vi "R=Peg_In_Hole_Jig.vi"(8 "Offset":T3, 9 "Matrix":T2 format="%.3f", 11 "Command":string="Load") -> (0 "error out":errorcluster, 2 "Joints":dbl[](array[numeric]), 3 "Pose Out":T2 format="%.3f")   [LabVIEW 2013]
uses:
  <vilib>/Analysis/Matrix/Datatypes/RealMatrix.ctl
  ROS/Code/SubVIs/BaxterSide.ctl
  ROS/Code/Console/Servers/ServerSubs/(nist) Arm Globals.vi
  <vilib>/Utility/config.llb/Read Key (String).vi
  Arm Globals.vi
  <vilib>/Analysis/baseanly.llb/Real Inverse Matrix.vi
  <vilib>/Analysis/Matrix/Numeric/Multiply/Multiply - RM,RM.vi
  <vilib>/Analysis/Matrix/Numeric/Conversions/Array To Matrix - RA.vi
  <vilib>/Utility/config.llb/Write Key (String).vi
  <vilib>/Analysis/NI_AALBase.lvlib
  <vilib>/Analysis/Matrix/NI_Matrix.lvlib
  <vilib>/Utility/config.llb/NI_LVConfig.lvlib
panel:
  in  "Tab Control":T1(tab)=enum."Calibration Table"
  out "IK Found":bool=TRUE
  in  "Table":dbl[][](array[numeric])
  in  "Reference":dbl[](array[numeric])=[40.0, -60.0, 0.0, 65.0, 0.0, 70.0, 0.0]
  # "Basic Commands are:\n   Convert   - convert offset to joints\n   Current   - current joint and offset\n   Save      - save calibration data\n   Load      - load calibration data\n   Reference - give reference joint position"
  # "Object X       ObjectY         ObjectZ        ObjectA         BaseX           BaseY           BaseZ          BaseA"
  # "Far Left"
  # "Far Right"
  # "Near Left"
  # "Near Right"
  # "Create cfg file to maintain \ncalibration data.\n\nThese values are loaded from there."
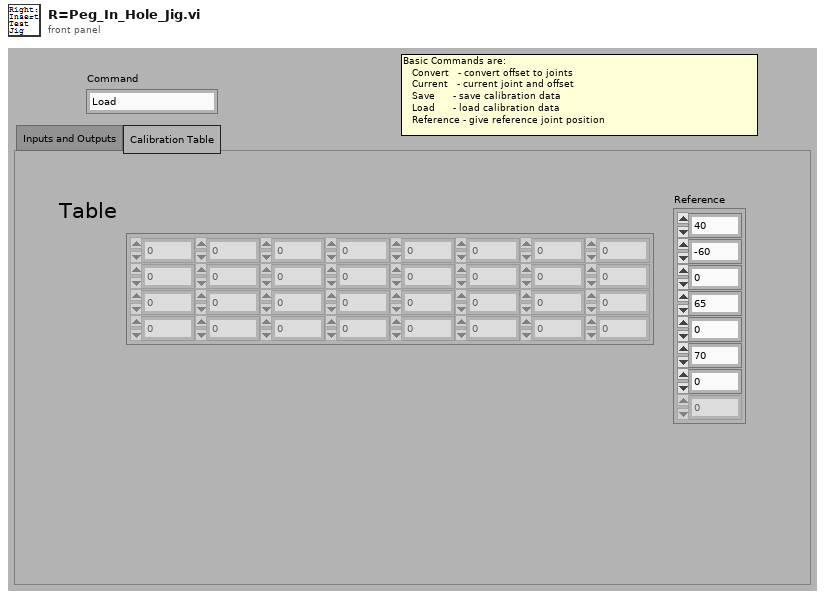
[diagram p1: front panel]
types:
  T1 = enum32{"Inputs and Outputs", "Calibration Table"}
  T2 = typedef "NI_Matrix.lvlib/RealMatrix.ctl" = dbl[][]
  T3 = cluster{"X":dbl, "Y":dbl, "Z":dbl, "Roll":dbl, "Pitch":dbl, "Yaw":dbl}
  T4 = typedef "BaxterSide.ctl" = enum16{"left", "right"}
  T5 = typedef "NI_LVConfig.lvlib/Config Data RefNum.ctl" = refnum<k1>
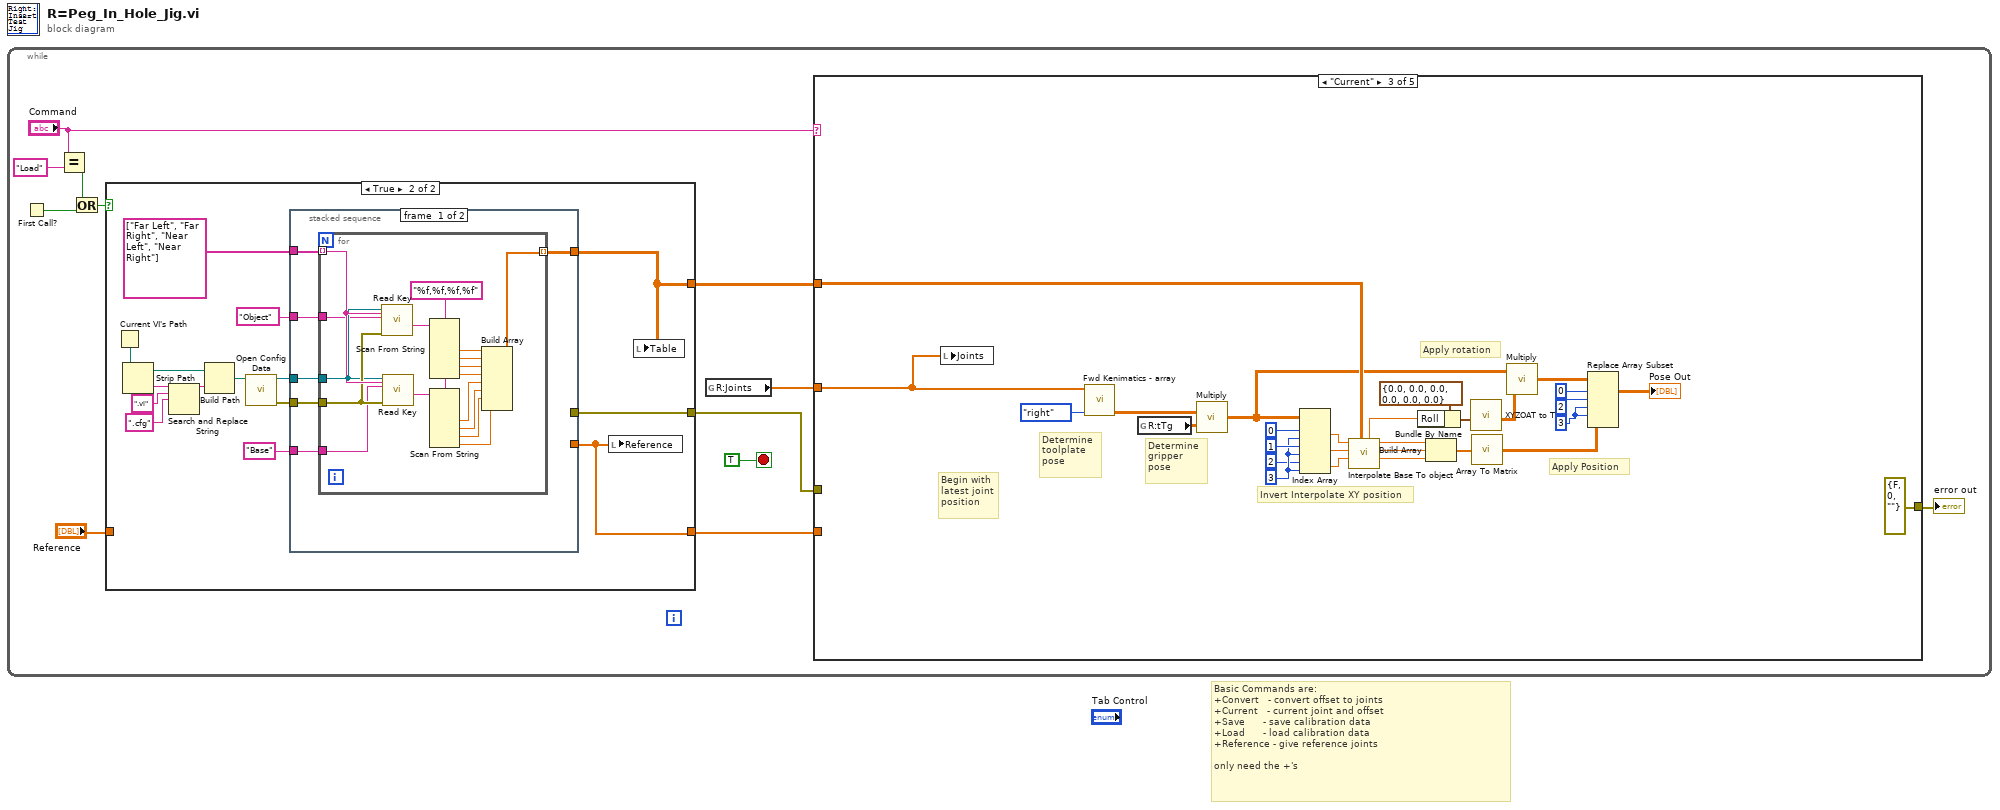
[diagram p0: block diagram]
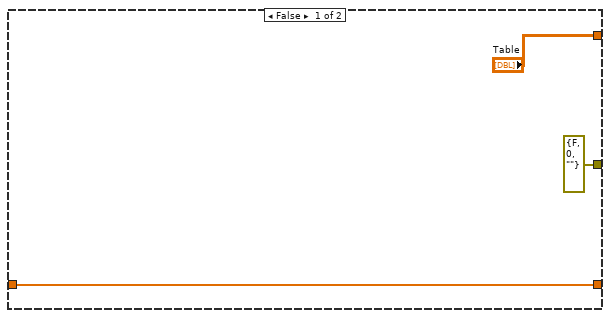
[diagram p2: hidden frame]
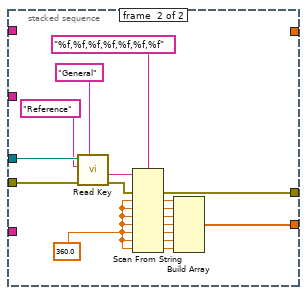
[diagram p3: hidden frame]
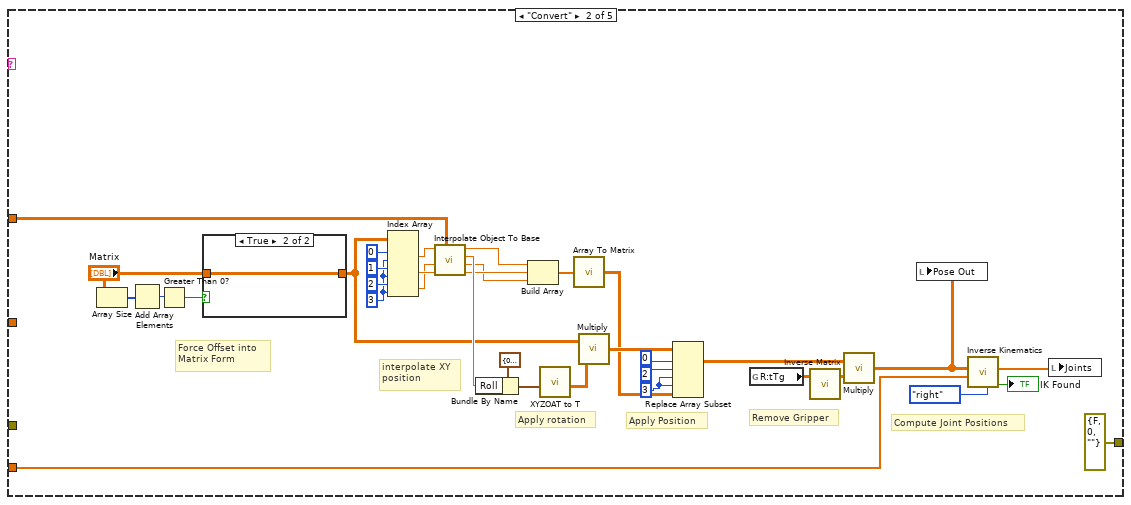
[diagram p5: hidden frame]
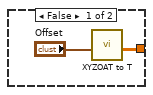
[diagram p6: hidden frame]
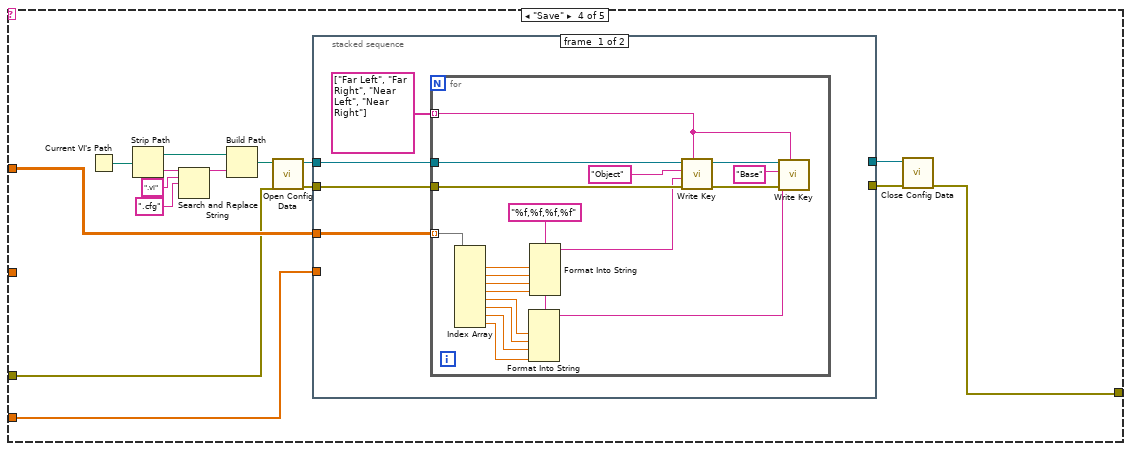
[diagram p7: hidden frame]
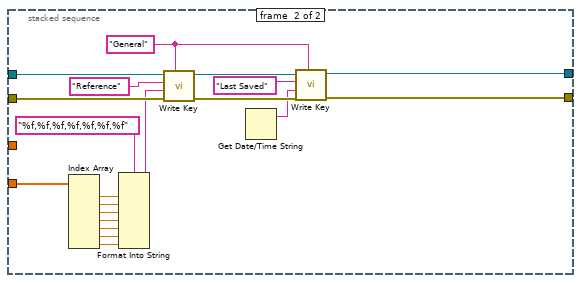
[diagram p8: hidden frame]
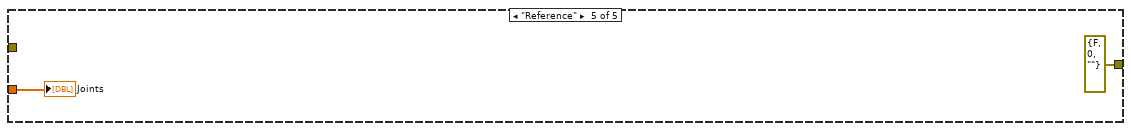
[diagram p9: hidden frame]
diagram:
  # "Basic Commands are:\n+Convert   - convert offset to joints\n+Current   - current joint and offset\n+Save      - save calibration data\n+Load      - load calibration data\n+Reference - give reference joints\n\nonly need the +'s"
  n1 = while {
    stop <- TRUE stop-if-true
    n2 = First Call?() -> (First Call?: T/F=w6:bool)
    n3 = Equal?(x="Command", y="Load") -> (x = y?=w7:bool)
    n4 = Or(x=w7, y=w6) -> (x .or. y?=w5:bool)
    n5 = case shown="True" w5 {
      tunnel: [errorcluster {"status"=FALSE, "code"=0, "source"=""} ("error IO") w19] -> w3
      tunnel: ["Table" w16] -> w4
      tunnel: "Reference" -> [w14 _]
      tunnel: [w14 w18] -> w1
      frame False {
      }
      frame True {
        n6 = Current VI's Path() -> (path=w28:path)
        n7 = Strip Path(path=w28) -> (stripped path=w23:path, name=w27:string)
        n8 = Search and Replace String(input string=w27, search string=".vi", replace string=".cfg" ("replace string (\"\")")) -> (result string=w24:string)  [unwired: 5 in, 3 out]
        n9 = Build Path(base path=w23, name or relative path=w24) -> (appended path=w22:path)
        n10 = call <vilib>:"Open Config Data.vi"("configuration file path"=w22) -> ("error out"=w29:errorcluster, "refnum"=w30:T5)  [unwired: 8 in, 1 out]
        n11 = stacked-sequence {
          tunnel: w30 -> [w35 w70]
          tunnel: w29 -> [w36 w69]
          tunnel: [_ w57] -> w18
          tunnel: "Object" ("key") -> [w34 _]
          tunnel: "Base" ("key") -> [w33 _]
          tunnel: [_ w54] -> w19
          tunnel: string[] ["Far Left", "Far Right", "Near Left", "Near Right"] -> [w32 _]
          tunnel: [w31 _] -> w16
          frame #0 {
            n12 = for {
              tunnel: w32 -> [w50] mode=indexing
              tunnel: w36 -> [w49]
              tunnel: w35 -> [w48]
              tunnel: w34 -> [w47]
              tunnel: w33 -> [w46]
              tunnel: [w44] -> w31 mode=indexing
              w52 = "%f,%f,%f,%f" ("format string")
              n13 = call-poly <vilib>:"Read Key.vi"("section"=w50, "error in (no error)"=w49, "key"=w47, "refnum"=w48) -> ("value"=w53:string)  [unwired: 4 in, 3 out]
              n14 = call-poly <vilib>:"Read Key.vi"("section"=w50, "error in (no error)"=w49, "key"=w46, "refnum"=w48) -> ("value"=w51:string)  [unwired: 4 in, 3 out]
              n15 = Scan From String(format string=w52, input string=w53) -> (output 1=w45:dbl, output 2=w43:dbl, output 3=w42:dbl, output 4=w41:dbl)  [unwired: 6 in, 3 out]
              n16 = Scan From String(format string=w52, input string=w51) -> (output 1=w40:dbl, output 2=w39:dbl, output 3=w38:dbl, output 4=w37:dbl)  [unwired: 6 in, 3 out]
              n17 = Build Array(w45, w43, w42, w41, w40, w39, w38, w37) -> (w44:dbl[])
            }
          }
          frame #1 {
            w56 = 360.0 ("default value 1")
            n18 = call-poly <vilib>:"Read Key.vi"("section"="General", "error in (no error)"=w69, "key"="Reference", "refnum"=w70) -> ("error out"=w55:errorcluster, "value"=w67:string)  [unwired: 4 in, 2 out]
            n19 = Scan From String(format string="%f,%f,%f,%f,%f,%f,%f", input string=w67, error in=w55, default 1=w56, default 2=w56, default 3=w56, default 4=w56, default 5=w56, default 6=w56, default 7=w56) -> (error out=w54:errorcluster, output 1=w66:dbl, output 2=w65:dbl, output 3=w64:dbl, output 4=w63:dbl, output 5=w60:dbl, output 6=w59:dbl, output 7=w58:dbl)  [unwired: 1 in, 2 out]
            n20 = Build Array(w66, w65, w64, w63, w60, w59, w58) -> (w57:dbl[])
          }
        }
        n21 = local write "Reference"(w18) -> ()
        n22 = local write "Table"(w16) -> ()
      }
    }
    n23 = global read "(nist) Arm Globals.vi" "R:Joints"() -> (w11:dbl[])
    n24 = case shown="\"Current\"" "Command" {
      tunnel: w4 -> [_ w92 w120 w142 _]
      tunnel: w1 -> [_ w76 _ w143 w197]
      tunnel: w11 -> [_ _ w119 _ _]
      tunnel: [w71 errorcluster {"status"=FALSE, "code"=0, "source"=""} ("error out") errorcluster {"status"=FALSE, "code"=0, "source"=""} ("error out") w141 errorcluster {"status"=FALSE, "code"=0, "source"=""} ("error out")] -> w10
      tunnel: w3 -> [w71 _ _ w138 _]
      frame Default {
      }
      frame "Convert" {
        w85 = 3 ("index (row)")
        w103 = 3 ("index (col)")
        # "Apply Position"
        # "Compute Joint Positions"
        # "Remove Gripper"
        # "Apply rotation"
        # "interpolate XY \nposition"
        # "Force Offset into \nMatrix Form"
        n25 = Array Size(array="Matrix") -> (size(s)=w95:i32[])
        n26 = Add Array Elements(numeric array=w95) -> (sum=w96:i32)
        n27 = Greater Than 0?(x=w96) -> (x > 0?=w94:bool)
        n28 = case shown="True" w94 {
          tunnel: "Matrix" -> [_ w109]
          tunnel: [w107 w109] -> w91
          frame False {
            n29 = call "XYZOAT to T.vi"("XYZOAT"="Offset") -> ("T"=w107:T2)  [unwired: 10 in]
          }
          frame True {
          }
        }
        n30 = Index Array(array=w91, index (row) #1=0 ("index (row)"), index (col) #1=w103, index (row) #2=1 ("index (row)"), index (col) #2=w103, index (row) #3=2 ("index (row)"), index (col) #3=w103) -> (element #1=w74:dbl, element #2=w73:dbl, element #3=w72:dbl)
        n31 = call "Interpolate Object To Base.vi"("Table"=w92, "Y"=w73, "Z"=w72, "X"=w74) -> ("y"=w83:dbl, "z"=w75:dbl, "a"=w100:dbl, "x"=w84:dbl)  [unwired: 4 in]
        n32 = Bundle By Name(cluster=T3 {"X"=0.0, "Y"=0.0, "Z"=0.0, "Roll"=0.0, "Pitch"=0.0, "Yaw"=0.0} ("XYZOAT"), "Roll"=w100) -> (w101:T3)
        n33 = Build Array(w84, w83, w75) -> (w82:dbl[])
        n34 = call "XYZOAT to T.vi"("XYZOAT"=w101) -> ("T"=w90:T2)  [unwired: 10 in]
        n35 = call-poly <vilib>:"Array To Matrix.vi"("Real 1D Array"=w82) -> ("Real Matrix (Column Vector)"=w81:T2)
        n36 = call-poly <vilib>:"Multiply.vi"("Real Matrix B"=w90, "Real Matrix A"=w91) -> ("A * B"=w89:T2)
        n37 = Replace Array Subset(array=w89, new element=w81, index (dim 0)=0 ("index (row)"), index (dim 1)=2 ("index (row)"), index (dim 2)=w85, index (dim 3)=w85) -> (w88:T2)
        n38 = global read "Arm Globals.vi" "R:tTg"() -> (w98:T2)
        n39 = call-poly <vilib>:"Inverse Matrix.vi"("Input Matrix"=w98) -> ("Inverse Matrix"=w99:T2)  [unwired: 1 in, 1 out]
        n40 = call-poly <vilib>:"Multiply.vi"("Real Matrix B"=w99, "Real Matrix A"=w88) -> ("A * B"=w77:T2)
        n41 = local write "Pose Out"(w77) -> ()
        n42 = call "Inverse Kinematics.vi"("Side"=BaxterSide."right", "Start"=w76, "Goal-matrix"=w77) -> ("Found"=→"IK Found":bool, "J"=w97:dbl[])  [unwired: 5 in, 2 out]
        n43 = local write "Joints"(w97) -> ()
      }
      frame "Current" {
        w123 = 3 ("index (row)")
        w133 = 3 ("index (col)")
        # "Apply Position"
        # "Apply rotation"
        # "Invert Interpolate XY position"
        # "Determine \ngripper\npose"
        # "Determine \ntoolplate\npose"
        # "Begin with\nlatest joint\nposition"
        n44 = local write "Joints"(w119) -> ()
        n45 = call "Fwd Kenimatics - array.vi"("Side"=BaxterSide."right", "Joints"=w119) -> ("Matrix"=w117:T2)  [unwired: 8 in, 1 out]
        n46 = global read "Arm Globals.vi" "R:tTg"() -> (w136:T2)
        n47 = call-poly <vilib>:"Multiply.vi"("Real Matrix B"=w136, "Real Matrix A"=w117) -> ("A * B"=w116:T2)
        n48 = Index Array(array=w116, index (row) #1=0 ("index (row)"), index (col) #1=w133, index (row) #2=1 ("index (row)"), index (col) #2=w133, index (row) #3=2 ("index (col)"), index (col) #3=w133) -> (element #1=w114:dbl, element #2=w113:dbl, element #3=w112:dbl)
        n49 = call "Interpolate Base To object.vi"("Table"=w120, "Z"=w112, "Y"=w113, "X"=w114) -> ("z"=w111:dbl, "y"=w127:dbl, "x"=w128:dbl, "a"=w110:dbl)  [unwired: 4 in]
        n50 = Bundle By Name(cluster=T3 {"X"=0.0, "Y"=0.0, "Z"=0.0, "Roll"=0.0, "Pitch"=0.0, "Yaw"=0.0} ("XYZOAT"), "Roll"=w110) -> (w130:T3)
        n51 = Build Array(w128, w127, w111) -> (w129:dbl[])
        n52 = call "XYZOAT to T.vi"("XYZOAT"=w130) -> ("T"=w126:T2)  [unwired: 10 in]
        n53 = call-poly <vilib>:"Array To Matrix.vi"("Real 1D Array"=w129) -> ("Real Matrix (Column Vector)"=w121:T2)
        n54 = call-poly <vilib>:"Multiply.vi"("Real Matrix B"=w126, "Real Matrix A"=w116) -> ("A * B"=w122:T2)
        n55 = Replace Array Subset(array=w122, new element=w121, index (dim 0)=0 ("index (row)"), index (dim 1)=2 ("index (row)"), index (dim 2)=w123, index (dim 3)=w123) -> (→"Pose Out":T2)
      }
      frame "Save" {
        n56 = Current VI's Path() -> (path=w150:path)
        n57 = Strip Path(path=w150) -> (stripped path=w145:path, name=w149:string)
        n58 = Search and Replace String(input string=w149, search string=".vi", replace string=".cfg" ("replace string (\"\")")) -> (result string=w146:string)  [unwired: 5 in, 3 out]
        n59 = Build Path(base path=w145, name or relative path=w146) -> (appended path=w144:path)
        n60 = call <vilib>:"Open Config Data.vi"("error in (no error)"=w138, "configuration file path"=w144) -> ("error out"=w151:errorcluster, "refnum"=w152:T5)  [unwired: 7 in, 1 out]
        n61 = stacked-sequence {
          tunnel: w152 -> [w156 w195]
          tunnel: w151 -> [w155 w194]
          tunnel: w142 -> [w154 _]
          tunnel: w143 -> [_ w191]
          tunnel: [_ w177] -> w140
          tunnel: [_ w176] -> w139
          frame #0 {
            n62 = for {
              tunnel: w156 -> [w175]
              tunnel: w155 -> [w174]
              tunnel: w154 -> [w158] mode=indexing
              tunnel: string[] ["Far Left", "Far Right", "Near Left", "Near Right"] -> [w157] mode=indexing
              w168 = "%f,%f,%f,%f" ("format string")
              n63 = Index Array(array=w158) -> (element #1=w166:dbl, element #2=w165:dbl, element #3=w164:dbl, element #4=w163:dbl, element #5=w162:dbl, element #6=w161:dbl, element #7=w160:dbl, element #8=w159:dbl)  [unwired: 8 in]
              n64 = Format Into String(format string=w168, w162, w161, w160, w159) -> (resulting string=w167:string)  [unwired: 2 in, 1 out]
              n65 = Format Into String(format string=w168, w166, w165, w164, w163) -> (resulting string=w172:string)  [unwired: 2 in, 1 out]
              n66 = call-poly <vilib>:"Write Key.vi"("section"=w157, "error in (no error)"=w174, "value"=w172, "key"="Object", "refnum"=w175) -> ("error out"=w170:errorcluster, "refnum out"=w171:T5)  [unwired: 4 in, 1 out]
              n67 = call-poly <vilib>:"Write Key.vi"("section"=w157, "error in (no error)"=w170, "value"=w167, "key"="Base", "refnum"=w171) -> ()  [unwired: 4 in, 3 out]
            }
          }
          frame #1 {
            w180 = "General" ("section")
            n68 = Index Array(array=w191) -> (element #1=w190:dbl, element #2=w189:dbl, element #3=w188:dbl, element #4=w187:dbl, element #5=w186:dbl, element #6=w185:dbl, element #7=w184:dbl)  [unwired: 7 in]
            n69 = Format Into String(format string="%f,%f,%f,%f,%f,%f,%f", w190, w189, w188, w187, w186, w185, w184) -> (resulting string=w183:string)  [unwired: 2 in, 1 out]
            n70 = call-poly <vilib>:"Write Key.vi"("section"=w180, "error in (no error)"=w194, "value"=w183, "key"="Reference", "refnum"=w195) -> ("error out"=w181:errorcluster, "refnum out"=w182:T5)  [unwired: 4 in, 1 out]
            n71 = Get Date/Time String() -> (date string=w179:string)  [unwired: 3 in, 1 out]
            n72 = call-poly <vilib>:"Write Key.vi"("section"=w180, "error in (no error)"=w181, "value"=w179, "key"="Last Saved", "refnum"=w182) -> ("error out"=w177:errorcluster, "refnum out"=w176:T5)  [unwired: 4 in, 1 out]
          }
        }
        n73 = call <vilib>:"Close Config Data.vi"("error in (no error)"=w140, "refnum"=w139) -> ("error out"=w141:errorcluster)  [unwired: 8 in, 1 out]
      }
      frame "Reference" {
        "Joints" <- w197
      }
    }
    "error out" <- w10
  }
